vi "Determine Join Tables.vi"(10 "Types":refnum<class "Type.lvclass">[](array[class]), 11 "SQLite":refnum<class "SQLite.lvclass">) -> (0 "error out":errorcluster, 2 "Join Tables":T1[](array[typedef]))   [LabVIEW 2020, in "Conditum SQLite.lvlib" / "SQLite.lvclass"]
uses:
  SQLite.lvclass
  SQLite.lvclass/SQLite.ctl
  <vilib>/IlluminatedG/IG Conditum Base/Conditum/Columns/Relation/Relation.lvclass
  <vilib>/ErrorRing/Error Ring.xnode
  <vilib>/Utility/error.llb/Error Cluster From Error Code.vi
  <vilib>/IlluminatedG/IG Conditum Base/Conditum/Relation Mapping.ctl
  <vilib>/IlluminatedG/IG Conditum Base/Conditum/Conditum.lvlib
  Join Table.ctl
  <vilib>/IlluminatedG/IG Conditum Base/Conditum/Entity/Entity.lvclass
  <vilib>/IlluminatedG/IG Conditum Base/Conditum/Columns/Type/Type.lvclass
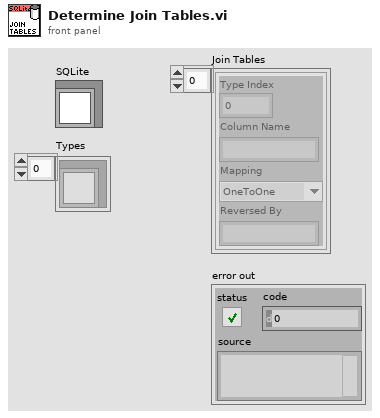
[diagram p1: front panel]
types:
  T1 = typedef "Conditum SQLite.lvlib/SQLite.lvclass/Join Table.ctl" = cluster{"Type Index":i32, "Column Name":string, "Mapping":T2, "Reversed By":string}
  T2 = typedef "Conditum.lvlib/Relation Mapping.ctl" = enum16{"OneToOne", "OneToMany", "ManyToOne", "ManyToMany"}
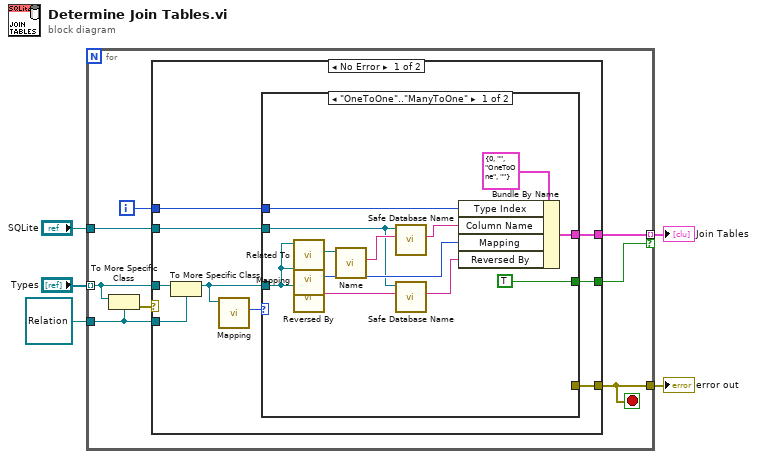
[diagram p0: block diagram]
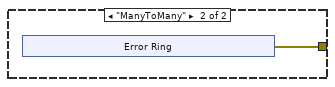
[diagram p2: hidden frame]
diagram:
  n1 = for {
    tunnel: "Types" -> [w12] mode=indexing
    tunnel: refnum<class "Relation.lvclass"> refnum ("Conditum:Columns:Relation.lvclass") -> [w11]
    tunnel: [w10] -> w3
    tunnel: "SQLite" -> [w9]
    tunnel: [w7] -> w1 mode=indexing if=w6
    i -> [w8]
    stop <- w10 stop-if-true
    n2 = To More Specific Class(target class=w11, reference=w12) -> (error out=w13:errorcluster)  [unwired: 1 in, 1 out]
    n3 = case shown="No Error" w13 {
      tunnel: w12 -> [w22 _]
      tunnel: w11 -> [w21 _]
      tunnel: [w19 _] -> w10
      tunnel: w9 -> [w17 _]
      tunnel: w8 -> [w16 _]
      tunnel: [w15 _] -> w7
      tunnel: [w14 _] -> w6
      frame No Error {
        n4 = To More Specific Class(target class=w21, reference=w22) -> (specific class reference=w18:refnum<class "Relation.lvclass">)  [unwired: 1 in, 1 out]
        n5 = call <vilib>:"Mapping.vi"("Relation in"=w18) -> ("Mapping"=w20:T2)  [unwired: 10 in]
        n6 = case shown="\"OneToOne\"..\"ManyToOne\"" w20 {
          tunnel: [_ w35] -> w19
          tunnel: w18 -> [w28 _]
          tunnel: w17 -> [w26 _]
          tunnel: w16 -> [w31 _]
          tunnel: [w24 _] -> w15
          tunnel: [TRUE _] -> w14
          frame "OneToOne".."ManyToOne" {
            n7 = call <vilib>:"Related To.vi"("Relation in"=w28) -> ("Related To"=w34:refnum<class "Entity.lvclass">)  [unwired: 9 in, 1 out]
            n8 = call <vilib>:"Mapping.vi"("Relation in"=w28) -> ("Mapping"=w29:T2)  [unwired: 10 in]
            n9 = call <vilib>:"Reversed By.vi"("Relation in"=w28) -> ("Reversed By"=w27:string)  [unwired: 10 in]
            n10 = call-dynamic "Name.vi"("Entity in"=w34) -> ("Name"=w33:string)  [unwired: 10 in]
            n11 = call-dynamic "Safe Database Name.vi"("Conditum Name"=w33, "Database in"=w26) -> ("Database Name"=w30:string)  [unwired: 9 in]
            n12 = call-dynamic "Safe Database Name.vi"("Conditum Name"=w27, "Database in"=w26) -> ("Database Name"=w25:string)  [unwired: 9 in]
            n13 = Bundle By Name(cluster=T1 {"Type Index"=0, "Column Name"="", "Mapping"=enum."OneToOne", "Reversed By"=""} ("Join Table"), "Type Index"=w31, "Column Name"=w30, "Mapping"=w29, "Reversed By"=w25) -> (w24:T1)
          }
          frame "ManyToMany" {
            n14 = xnode "Error Ring"() -> ("error out"=w35:errorcluster)
          }
        }
      }
      frame Error {
      }
    }
  }
  "error out" <- w3
  "Join Tables" <- w1
